vi "Main Brute Force.vi"   [LabVIEW 2020]
uses:
  <vilib>/DAQmx/create/channels.llb/DAQmx Create Channel (DO-Digital Output).vi
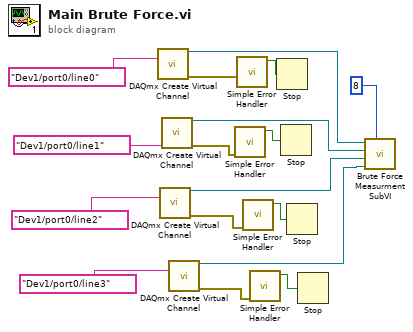
[diagram p0: block diagram]
diagram:
  n1 = call-poly <vilib>:"DAQmx Create Virtual Channel.vi"("lines"=tag "Dev1/port0/line0" ("Data Pin")) -> ("task out"=w13:refnum<k21>, "error out"=w8:errorcluster)  [unwired: 13 in]
  n2 = call-poly <vilib>:"DAQmx Create Virtual Channel.vi"("lines"=tag "Dev1/port0/line2" ("Write Pin")) -> ("task out"=w11:refnum<k21>, "error out"=w6:errorcluster)  [unwired: 13 in]
  n3 = call-poly <vilib>:"DAQmx Create Virtual Channel.vi"("lines"=tag "Dev1/port0/line1" ("Sync Pin")) -> ("task out"=w12:refnum<k21>, "error out"=w7:errorcluster)  [unwired: 13 in]
  n4 = call-poly <vilib>:"DAQmx Create Virtual Channel.vi"("lines"=tag "Dev1/port0/line3" ("Clear Pin")) -> ("task out"=w10:refnum<k21>, "error out"=w5:errorcluster)  [unwired: 13 in]
  n5 = call <vilib>:"Simple Error Handler.vi"("error in (no error)"=w7) -> ("error?"=w1:bool)  [unwired: 4 in, 4 out]
  n6 = call <vilib>:"Simple Error Handler.vi"("error in (no error)"=w8) -> ("error?"=w4:bool)  [unwired: 4 in, 4 out]
  n7 = call <vilib>:"Simple Error Handler.vi"("error in (no error)"=w6) -> ("error?"=w2:bool)  [unwired: 4 in, 4 out]
  n8 = call <vilib>:"Simple Error Handler.vi"("error in (no error)"=w5) -> ("error?"=w3:bool)  [unwired: 4 in, 4 out]
  n9 = Stop(stop? (T)=w4) -> ()
  n10 = Stop(stop? (T)=w1) -> ()
  n11 = Stop(stop? (T)=w2) -> ()
  n12 = Stop(stop? (T)=w3) -> ()
  n13 = call "Brute Force Measurment SubVI.vi"("Number of Active tubes"=8, "Clear Pin Task In"=w10, "Write Pin Task In"=w11, "Sync Pin Task In"=w12, "Data Pin Task In"=w13) -> ()  [unwired: 3 in, 4 out]
